vi "myRIO_BRig_Host_isExcelRunning.vi"() -> (2 "output_Iexcel":bool)   [LabVIEW 2014]
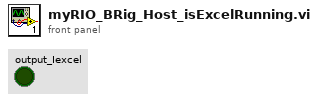
[diagram p1: front panel]
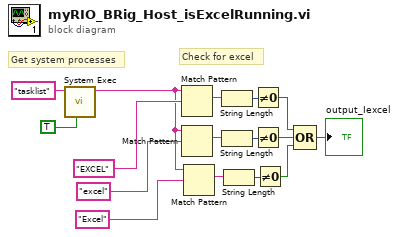
[diagram p0: block diagram]
diagram:
  # "Check for excel"
  # "Get system processes"
  n1 = call <vilib>:"System Exec.vi"("run minimized? (F)"=TRUE, "command line"="tasklist") -> ("standard output"=w7:string)  [unwired: 6 in, 3 out]
  n2 = Match Pattern(string=w7, regular expression="EXCEL" ("search string/char (-)")) -> (match substring=w13:string)  [unwired: 1 in, 3 out]
  n3 = Match Pattern(string=w7, regular expression="excel" ("search string/char (-)")) -> (match substring=w11:string)  [unwired: 1 in, 3 out]
  n4 = Match Pattern(string=w7, regular expression="Excel" ("search string/char (-)")) -> (match substring=w9:string)  [unwired: 1 in, 3 out]
  n5 = String Length(string=w13) -> (length=w12:i32)
  n6 = String Length(string=w11) -> (length=w10:i32)
  n7 = String Length(string=w9) -> (length=w8:i32)
  n8 = Not Equal To 0?(x=w12) -> (x != 0?=w6:bool)
  n9 = Not Equal To 0?(x=w10) -> (x != 0?=w5:bool)
  n10 = Not Equal To 0?(x=w8) -> (x != 0?=w4:bool)
  n11 = Compound Arithmetic op=OR(w6, w5, w4) -> (→"output_Iexcel":bool)
